vi "Send.vi"(7 "Ignore Network Down (T)":bool=TRUE, 8 "error in (no error)":errorcluster, 9 "Destination Location":T3, 10 "Send Data":string, 11 "UDP Base in":T1) -> (0 "error out":errorcluster, 3 "UDP Base out":T1, 6 "Comm Error":bool)   [LabVIEW 2011]
uses:
  UDP Network Location.ctl
  UDP Base.ctl
  UDP Socket Params.ctl
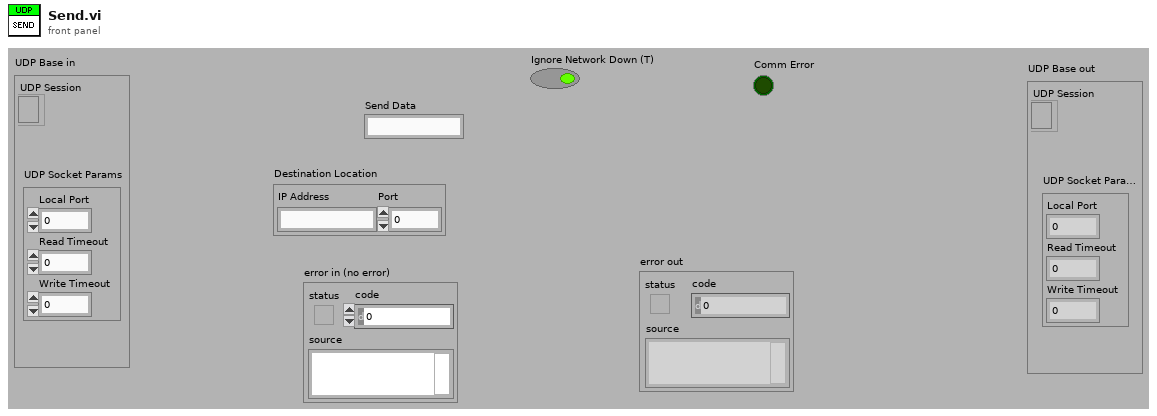
[diagram p1: front panel]
types:
  T1 = typedef "UDP Base.ctl" = cluster{"UDP Session":refnum<k16>, "UDP Socket Params":T2}
  T2 = typedef "UDP Socket Params.ctl" = cluster{"Local Port":u16, "Read Timeout":i32, "Write Timeout":i32}
  T3 = typedef "UDP Network Location.ctl" = cluster{"IP Address":string, "Port":u16}
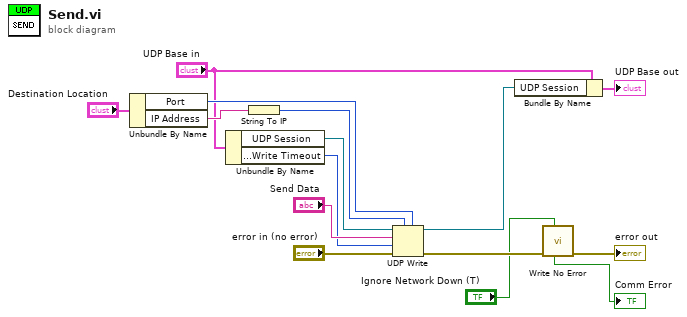
[diagram p0: block diagram]
diagram:
  n1 = Unbundle By Name("Destination Location") -> ("Port"=w7:u16, "IP Address"=w6:string)
  n2 = Unbundle By Name("UDP Base in") -> ("UDP Session"=w15:refnum<k16>, "UDP Socket Params.Write Timeout"=w1:i32)
  n3 = String To IP(1:w6) -> (0:w14:u32)
  n4 = UDP Write(address=w14, port or service name=w7, connection ID=w15, data in="Send Data", 8:"error in (no error)", 9:w1) -> (error out=w11:errorcluster, 3:w13:refnum<k16>)
  n5 = Bundle By Name(cluster="UDP Base in", "UDP Session"=w13) -> (→"UDP Base out":T1)
  n6 = call "Write No Error.vi"("Ignore Network Down"="Ignore Network Down (T)", "error in (no error)"=w11) -> ("error out"=→"error out":errorcluster, "Comm Error"=→"Comm Error":bool)  [unwired: 8 out]
